vi "Match Frequency Range.vi"(0 "VISA resource name":refnum<visa-resource-name>, 1 "Channel (1)":i32=1, 5 "Function (0: Time Domain)":u16(ring) items=["Time Domain", "Fault Location"], 11 "error in (no error)":errorcluster) -> (4 "VISA resource name out":refnum<visa-resource-name>, 15 "error out":errorcluster)   [LabVIEW 2012, in "Tektronix TTR500 Series.lvlib"]
doc: "For the active trace of selected channel, changes the frequency range to match with the low-pass type transformation of the transformation function of the time domain function."
uses:
  <instrlib>/Tektronix TTR500 Series/Tektronix TTR500 Series.lvlib
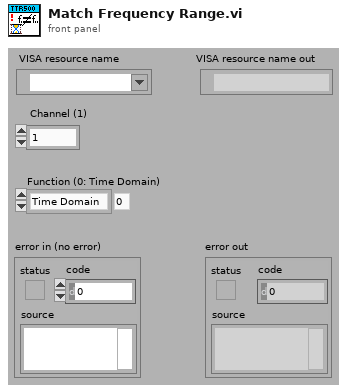
[diagram p1: front panel]
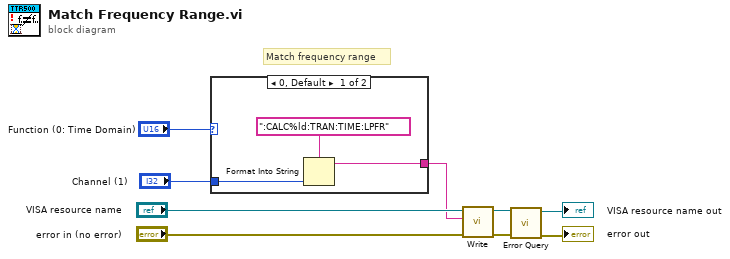
[diagram p0: block diagram]
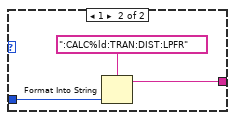
[diagram p2: hidden frame]
diagram:
  # "Match frequency range"
  n1 = case shown="0, Default" "Function (0: Time Domain)" {
    tunnel: "Channel (1)" -> [w11 w14]
    tunnel: [w10 w13] -> w6
    frame 0, Default {
      n2 = Format Into String(format string=":CALC%ld:TRAN:TIME:LPFR", w11) -> (resulting string=w10:string)  [unwired: 2 in, 1 out]
    }
    frame 1 {
      n3 = Format Into String(format string=":CALC%ld:TRAN:DIST:LPFR", w14) -> (resulting string=w13:string)  [unwired: 2 in, 1 out]
    }
  }
  n4 = call <instrlib>:"Write.vi"("error in (no error)"="error in (no error)", "String ()"=w6, "VISA resource name"="VISA resource name") -> ("error out"=w4:errorcluster, "VISA resource name out"=w5:refnum<visa-resource-name>)  [unwired: 6 in, 1 out]
  n5 = call <instrlib>:"Error Query.vi"("error in (no error)"=w4, "VISA resource name"=w5) -> ("error out"=→"error out":errorcluster, "VISA resource name out"=→"VISA resource name out":refnum<visa-resource-name>)  [unwired: 6 in, 2 out]
